vi "launch-daq-damon.vi"(8 "error in (no error)":errorcluster, 10 "Parameters":T1) -> (0 "error out":errorcluster, 3 "queue out":refnum<queue>)   [LabVIEW 2014]
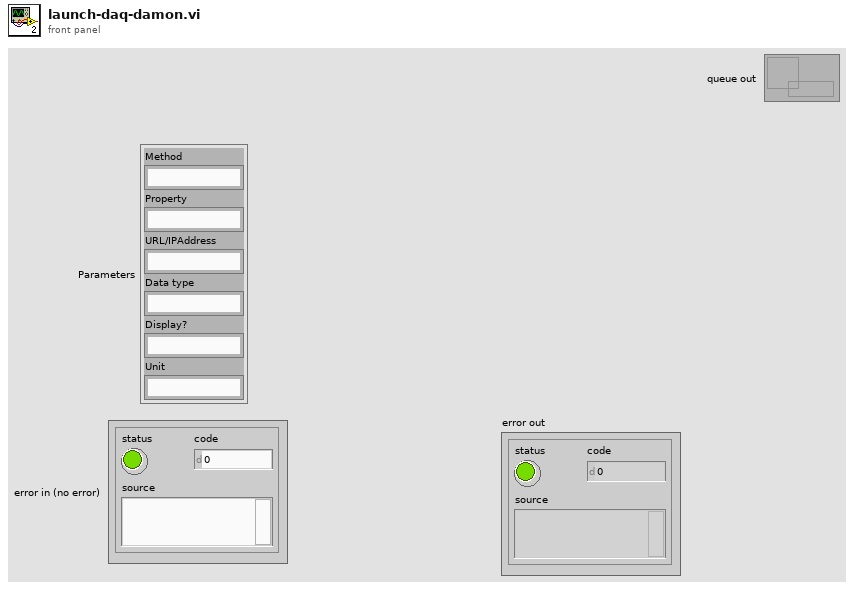
[diagram p1: front panel]
types:
  T1 = cluster{"Method":string, "Property":string, "URL/IPAddress":string, "Data type":string, "Display?":string, "Unit":string}
  T2 = cluster{"Method":string, "PropertyName":string, "Value":string, "Display?":string, "Unit":string}
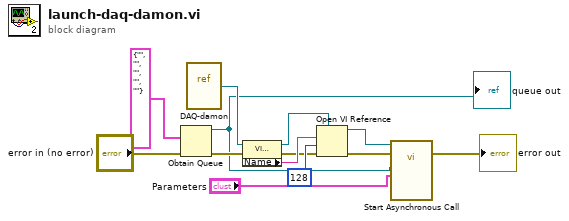
[diagram p0: block diagram]
diagram:
  n1 = Obtain Queue(element data type=T2 {"Method"="", "PropertyName"="", "Value"="", "Display?"="", "Unit"=""} ("DataPack"), error in (no error)="error in (no error)") -> (queue out=w1:refnum<queue>, error out=w4:errorcluster)  [unwired: 3 in, 1 out]
  "queue out" <- w1
  n2 = vi-ref "DAQ-damon.vi"() -> (w12:refnum<vi>)
  n3 = property class="VI (strict)"(reference=w12, error in=w4) -> (reference out=w11:refnum<vi>, error out=w3:errorcluster, "Name"=w10:string)
  n4 = Open VI Reference(type specifier VI Refnum (for type only)=w11, vi path=w10, options=128, error in (no error)=w3) -> (vi reference=w9:refnum<vi>, error out=w7:errorcluster)  [unwired: 2 in]
  n5 = call-by-ref "Start Asynchronous Call"(reference=w9, error in=w7, "Parameters"="Parameters", "queue out"=w1) -> (error out=→"error out":errorcluster)  [unwired: 10 in, 1 out]
